vi "weight_experimental3.vi"(9 "Stop read":bool, 10 "N_points":i32=4200, 11 "PV weight":dbl caption="g" format="%#.0f") -> (1 "Q3":dbl caption="mg/s" format="%#.0f", 2 "Q 1":dbl caption="mg/s" format="%#.0f", 3 "Weight 1":dbl caption="g" format="%#.0f", 5 "This VI":refnum<vi>)   [LabVIEW 2019]
uses:
  <vilib>/Analysis/baseanly.llb/Mean (DBL).vi
  Logik/fronts.vi
  Trigers/RS.vi
  <vilib>/Analysis/NI_AALBase.lvlib
  Timer Delay/Timers.lvlib
panel:
  in  "Tab Control":T1(tab)
  out "dM 3":dbl caption="g" format="%#.0f"
  out "dM 1":dbl caption="g" format="%#.0f"
  out "variance":dbl format="%0.2f"
  out "standard deviation":dbl format="%0.2f"
  in  "Tare":dbl caption="g" format="%#.0f"
  in  "<0>":bool
  in  "<вес>":bool
  in  "k":dbl=1.0 caption="g" format="%#.3f"
  in  "Вес":dbl caption="g" format="%#.0f"
  # "Усреднение за 1 мин"
  # "(расход)"
  # "Усреднение за 3 мин"
  # "(расход)"
  # "Вес тары\n(полностью очистить бункер от продукта\nи запомнить PV weight или ввести вручную)."
  # "Вес тары\n(ввести фактический вес без учета тары\nили ввести k вручную)"
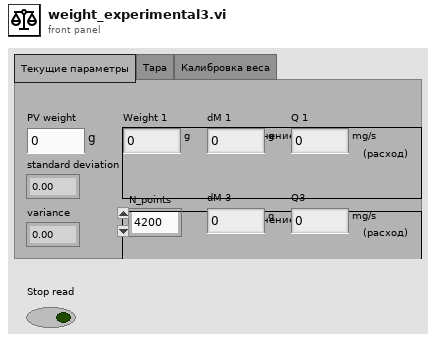
[diagram p1: front panel]
types:
  T1 = enum32{"Текущие параметры", "Тара", "Калибровка веса"}
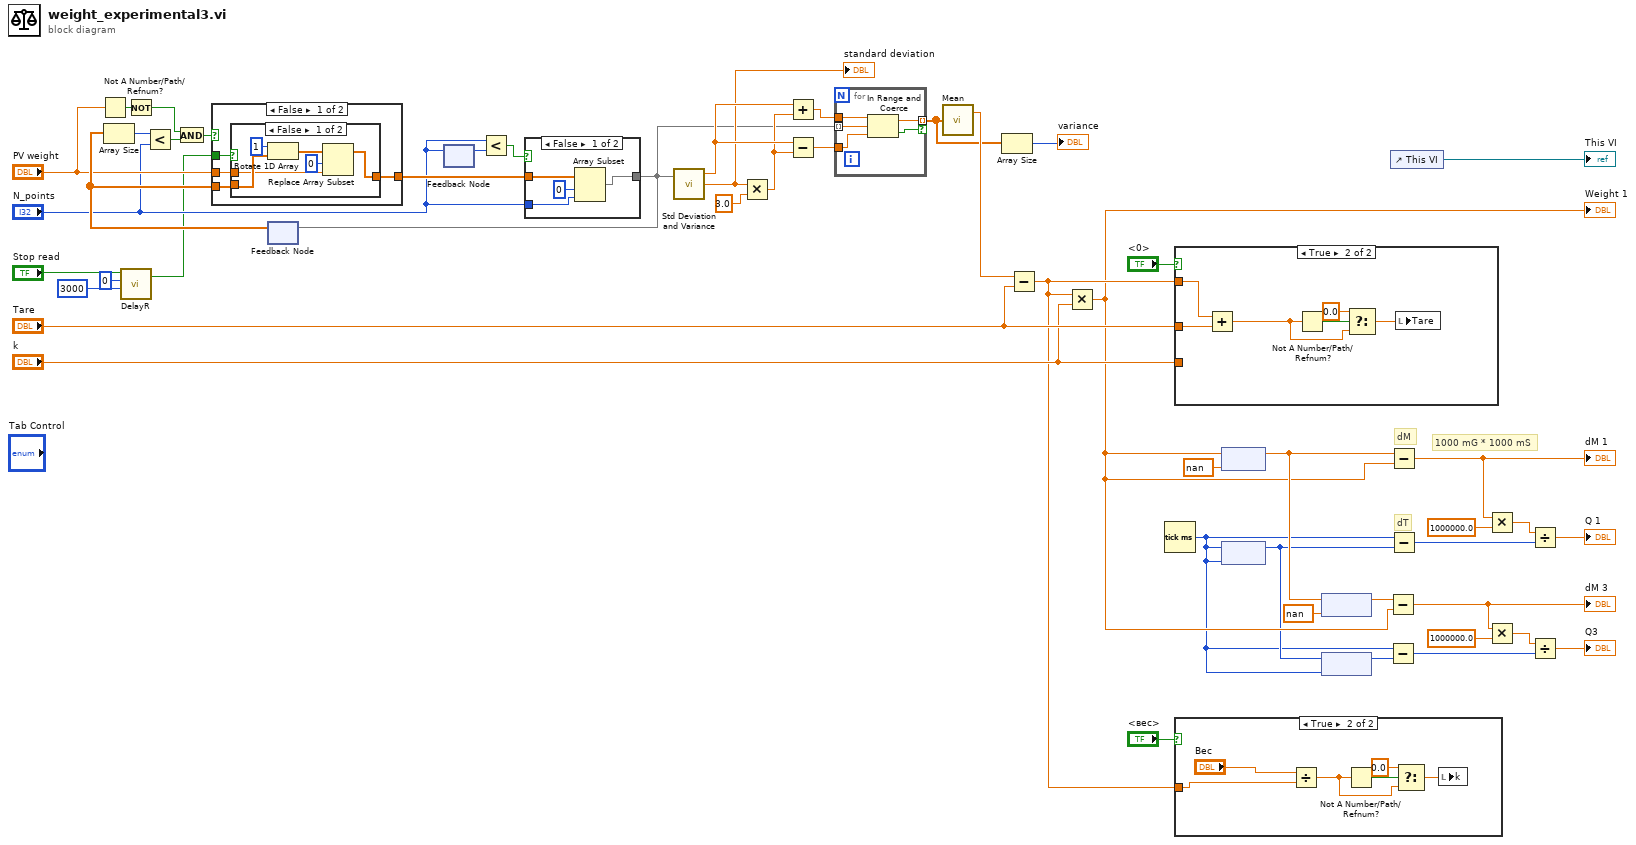
[diagram p0: block diagram]
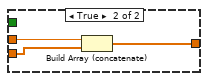
[diagram p4: hidden frame]
diagram:
  # "1000 mG * 1000 mS"
  # "dM"
  # "dT"
  n1 = Not A Number/Path/Refnum?(number/path/refnum="PV weight") -> (NaN/Path/Refnum?=w12:bool)
  n2 = call "DelayR.vi"("DelayOff"=u32 3000, "DelayOn"=u32 0, "In"="Stop read") -> ("Out"=w3:bool)  [unwired: 1 in, 1 out]
  n3 = Not(x=w12) -> (.not. x?=w10:bool)
  n4 = feedback #1() -> (w15:dbl[])  [unwired: 1 in]
  n5 = Array Size(array=w15) -> (size(s)=w16:i32)
  n6 = Less?(x=w16, y="N_points") -> (x < y?=w14:bool)
  n7 = And(x=w10, y=w14) -> (x .and. y?=w13:bool)
  n8 = case shown="False" w13 {
    tunnel: [w51 w62] -> w9
    tunnel: "PV weight" -> [w52 w63]
    tunnel: w15 -> [w53 w61]
    tunnel: w3 -> [w50 _]
    frame False {
      n9 = case shown="False" w50 {
        tunnel: w53 -> [w56 w60]
        tunnel: w52 -> [w55 _]
        tunnel: [w54 w60] -> w51
        frame False {
          n10 = Rotate 1D Array(1:w56, 2:1 ("n")) -> (0:w58:dbl[])
          n11 = Replace Array Subset(array=w58, new element=w55, index=0) -> (w54:dbl[])
        }
        frame True {
        }
      }
    }
    frame True {
      n12 = Build Array (concatenate)(w63, w61) -> (w62:dbl[])
    }
  }
  n13 = feedback #2() -> (w7:i32)  [unwired: 1 in]
  n14 = feedback-in #2("N_points") -> ()
  n15 = Less?(x="N_points", y=w7) -> (x < y?=w6:bool)
  n16 = case shown="False" w6 {
    tunnel: [w66 w68] -> w5
    tunnel: w9 -> [w67 w68]
    tunnel: "N_points" -> [w64 _]
    frame False {
      n17 = Array Subset(array=w67, index=0, length=w64) -> (w66:dbl[])
    }
    frame True {
    }
  }
  n18 = feedback-in #1(w5) -> ()
  n19 = call <vilib>:"Std Deviation and Variance.vi"("X"=w5) -> ("mean"=w25:dbl, "standard deviation"=w19:dbl)  [unwired: 1 in, 1 out]
  "standard deviation" <- w19
  n20 = Multiply(x=w19, y=3.0) -> (x*y=w17:dbl)
  n21 = Add(x=w25, y=w17) -> (x+y=w24:dbl)
  n22 = Subtract(x=w25, y=w17) -> (x-y=w23:dbl)
  n23 = for {
    tunnel: w5 -> [w71] mode=indexing
    tunnel: w24 -> [w73]
    tunnel: w23 -> [w72]
    tunnel: [w70] -> w20 mode=indexing if=w69
    n24 = In Range and Coerce(upper limit=w73, x=w71, lower limit=w72) -> (coerced(x)=w70:dbl, In Range?=w69:bool)
  }
  n25 = call-poly <vilib>:"Mean.vi"("X"=w20) -> ("mean"=w22:dbl)  [unwired: 1 out]
  n26 = Array Size(array=w20) -> (size(s)=→"variance":i32)
  n27 = Subtract(x=w22, y="Tare") -> (x-y=w36:dbl)
  n28 = Multiply(x=w36, y="k") -> (x*y=w34:dbl)
  "Weight 1" <- w34
  n29 = Tick Count (ms)() -> (millisecond timer value=w31:u32)
  n30 = case shown="True" "<0>" {
    tunnel: "Tare" -> [_ w76]
    tunnel: w36 -> [_ w75]
    tunnel: "k" -> [_ _]
    frame False {
    }
    frame True {
      n31 = Add(x=w75, y=w76) -> (x+y=w74:dbl)
      n32 = Not A Number/Path/Refnum?(number/path/refnum=w74) -> (NaN/Path/Refnum?=w79:bool)
      n33 = Select(t=0.0 ("y"), s=w79, f=w74) -> (s? t:f=w77:dbl)
      n34 = local write "Tare"(w77) -> ()
    }
  }
  n35 = case shown="True" "<вес>" {
    tunnel: w36 -> [_ w80]
    frame False {
    }
    frame True {
      n36 = Divide(x="Вес", y=w80) -> (x/y=w83:dbl)
      n37 = Not A Number/Path/Refnum?(number/path/refnum=w83) -> (NaN/Path/Refnum?=w85:bool)
      n38 = Select(t=0.0 ("y"), s=w85, f=w83) -> (s? t:f=w82:dbl)
      n39 = local write "k"(w82) -> ()
    }
  }
  n40 = feedback #3(nan) -> (w45:dbl)
  n41 = feedback-in #3(w34) -> ()
  n42 = feedback #4(w31) -> (w33:u32)
  n43 = feedback-in #4(w31) -> ()
  n44 = feedback #5(nan) -> (w46:dbl)
  n45 = feedback-in #5(w45) -> ()
  n46 = feedback #6(w31) -> (w32:u32)
  n47 = feedback-in #6(w33) -> ()
  n48 = Subtract(x=w46, y=w34) -> (x-y=w27:dbl)
  "dM 3" <- w27
  n49 = Subtract(x=w31, y=w32) -> (x-y=w28:u32)
  n50 = Subtract(x=w45, y=w34) -> (x-y=w40:dbl)
  "dM 1" <- w40
  n51 = Subtract(x=w31, y=w33) -> (x-y=w38:u32)
  n52 = control-ref of="This VI"() -> (→"This VI":refnum<vi>)
  n53 = Multiply(x=w40, y=1000000.0) -> (x*y=w39:dbl)
  n54 = Multiply(x=w27, y=1000000.0) -> (x*y=w30:dbl)
  n55 = Divide(x=w39, y=w38) -> (x/y=→"Q 1":dbl)
  n56 = Divide(x=w30, y=w28) -> (x/y=→"Q3":dbl)
